vi "Q -- range multiplier -- real -- V2.vi"(6 "factor":dbl=1.1, 7 "rage multiplier action":T1=enum."zoom", 8 "center":dbl=nan, 9 "window":dbl=nan, 10 "lower":dbl=nan, 11 "upper":dbl=nan) -> (0 "center OUT":dbl, 1 "window OUT":dbl, 2 "lower OUT":dbl, 3 "upper OUT":dbl)   [LabVIEW 2021]
uses:
  range multiplier action.ctl
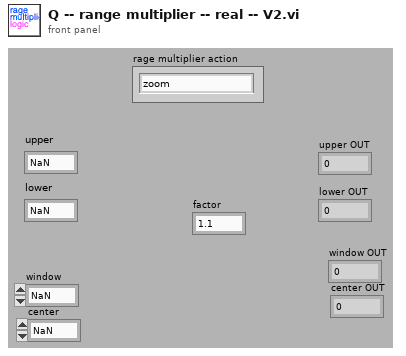
[diagram p1: front panel]
types:
  T1 = typedef "range multiplier action.ctl" = enum16{"shift", "zoom", "check"}
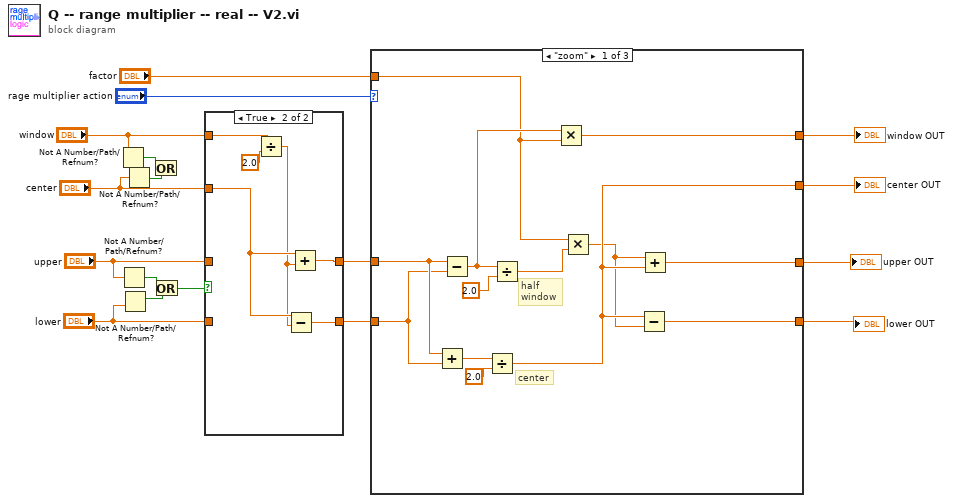
[diagram p0: block diagram]
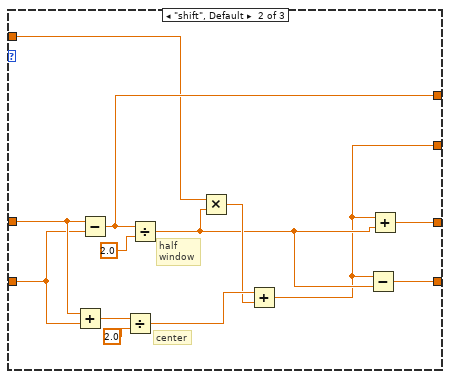
[diagram p3: hidden frame]
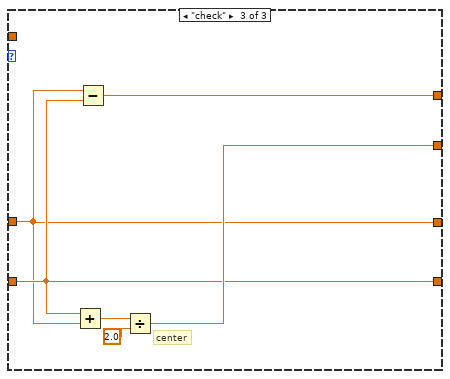
[diagram p4: hidden frame]
diagram:
  n1 = Not A Number/Path/Refnum?(number/path/refnum="window") -> (NaN/Path/Refnum?=w11:bool)
  n2 = Not A Number/Path/Refnum?(number/path/refnum="upper") -> (NaN/Path/Refnum?=w8:bool)
  n3 = Not A Number/Path/Refnum?(number/path/refnum="lower") -> (NaN/Path/Refnum?=w9:bool)
  n4 = Not A Number/Path/Refnum?(number/path/refnum="center") -> (NaN/Path/Refnum?=w10:bool)
  n5 = Or(x=w11, y=w10) -> ()  [unwired: 1 out]
  n6 = Or(x=w8, y=w9) -> (x .or. y?=w7:bool)
  n7 = case shown="True" w7 {
    tunnel: [w19 w23] -> w6
    tunnel: "upper" -> [w19 _]
    tunnel: [w18 w22] -> w4
    tunnel: "lower" -> [w18 _]
    tunnel: "window" -> [_ w24]
    tunnel: "center" -> [_ w21]
    frame False {
    }
    frame True {
      n8 = Divide(x=w24, y=2.0) -> (x/y=w20:dbl)
      n9 = Subtract(x=w21, y=w20) -> (x-y=w22:dbl)
      n10 = Add(x=w21, y=w20) -> (x+y=w23:dbl)
    }
  }
  n11 = case shown="\"zoom\"" "rage multiplier action" {
    tunnel: [w26 w50 w57] -> w17
    tunnel: "factor" -> [w27 w49 _]
    tunnel: w6 -> [w35 w46 w52]
    tunnel: w4 -> [w34 w45 w53]
    tunnel: [w32 w39 w54] -> w15
    tunnel: [w30 w44 w52] -> w14
    tunnel: [w29 w43 w53] -> w13
    frame "zoom" {
      # "half\nwindow"
      # "center"
      n12 = Add(x=w35, y=w34) -> (x+y=w36:dbl)
      n13 = Subtract(x=w35, y=w34) -> (x-y=w28:dbl)
      n14 = Divide(x=w36, y=2.0) -> (x/y=w32:dbl)
      n15 = Divide(x=w28, y=2.0) -> (x/y=w33:dbl)
      n16 = Multiply(x=w28, y=w27) -> (x*y=w26:dbl)
      n17 = Multiply(x=w27, y=w33) -> (x*y=w31:dbl)
      n18 = Subtract(x=w32, y=w31) -> (x-y=w29:dbl)
      n19 = Add(x=w31, y=w32) -> (x+y=w30:dbl)
    }
    frame "shift", Default {
      # "half\nwindow"
      # "center"
      n20 = Add(x=w46, y=w45) -> (x+y=w47:dbl)
      n21 = Subtract(x=w46, y=w45) -> (x-y=w50:dbl)
      n22 = Divide(x=w47, y=2.0) -> (x/y=w42:dbl)
      n23 = Divide(x=w50, y=2.0) -> (x/y=w40:dbl)
      n24 = Multiply(x=w49, y=w40) -> (x*y=w41:dbl)
      n25 = Add(x=w42, y=w41) -> (x+y=w39:dbl)
      n26 = Subtract(x=w39, y=w40) -> (x-y=w43:dbl)
      n27 = Add(x=w39, y=w40) -> (x+y=w44:dbl)
    }
    frame "check" {
      # "center"
      n28 = Add(x=w53, y=w52) -> (x+y=w55:dbl)
      n29 = Subtract(x=w52, y=w53) -> (x-y=w57:dbl)
      n30 = Divide(x=w55, y=2.0) -> (x/y=w54:dbl)
    }
  }
  "upper OUT" <- w14
  "lower OUT" <- w13
  "window OUT" <- w17
  "center OUT" <- w15
